vi "signalAnalysis.vi"(8 "error in (no error)":errorcluster, 9 "inpuPara":T1={"Rising[%] 1"=63.0, "Rising[%] 2"=99.0, "Falling[%]"=37.0}, 10 "data_scope":waveform(dbl), 11 "출력 전압 전류 특성":waveform(dbl)[](graph)=[{"t0"=timestamp(0 s since 1904-01-01), "dt"=0.0002, "Y"=array[10001 elements]}, {"t0"=timestamp(0 s since 1904-01-01), "dt"=0.0002, "Y"=array[10001 elements]}]) -> (0 "error out":errorcluster, 3 "data":T2)   [LabVIEW 2019]
uses:
  <vilib>/measure/mascope.llb/Transition Measurements 1 chan.vi
  <vilib>/measure/mascope.llb/Cycle Average and RMS 1 chan.vi
  <vilib>/measure/NI_MAPro.lvlib
panel:
  out "전체 저항 변화 2":waveform(dbl)(graph)
  out "measurement info":T3 {"ref levels"."ref units" items=["absolute", "relative"]; "ref levels"."high ref level" format="%.2p"; "ref levels"."low ref level" format="%.2p"; "ref levels"."mid ref level" format="%.2p"; "end time" format="%.2p"; "start time" format="%.2p"}
  out "접촉저항 변화":dbl[](graph)
  out "접촉 시 전압 변화":waveform(dbl)(graph)
  out "전체 저항 변화":dbl[](graph)
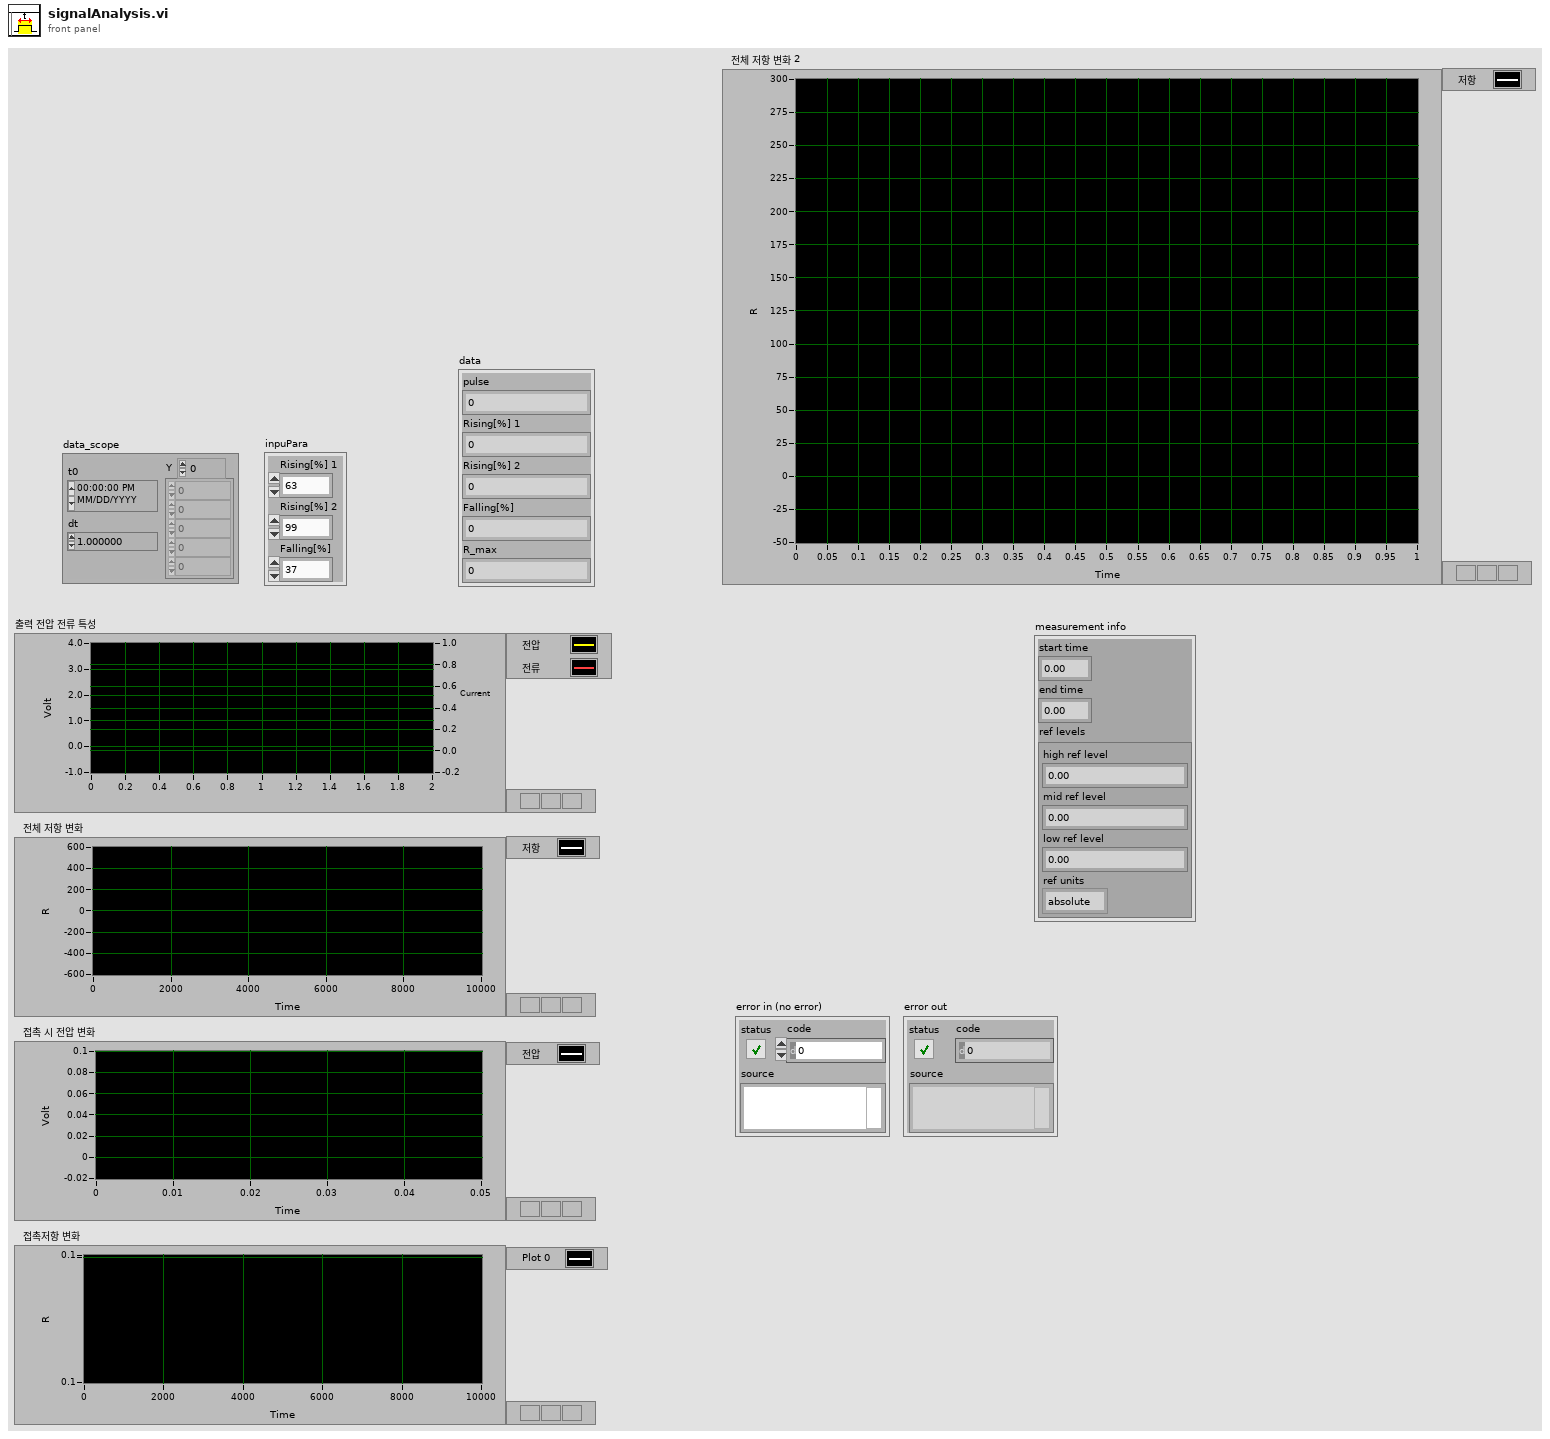
[diagram p1: front panel]
types:
  T1 = cluster{"Rising[%] 1":dbl, "Rising[%] 2":dbl, "Falling[%]":dbl}
  T2 = cluster{"pulse":i32, "Rising[%] 1":dbl, "Rising[%] 2":dbl, "Falling[%]":dbl, "R_max":dbl}
  T3 = cluster{"start time":dbl, "end time":dbl, "ref levels":cluster{"high ref level":dbl, "mid ref level":dbl, "low ref level":dbl, "ref units":u16}}
  T4 = cluster{"high ref level":dbl, "mid ref level":dbl, "low ref level":dbl, "ref units":u16}
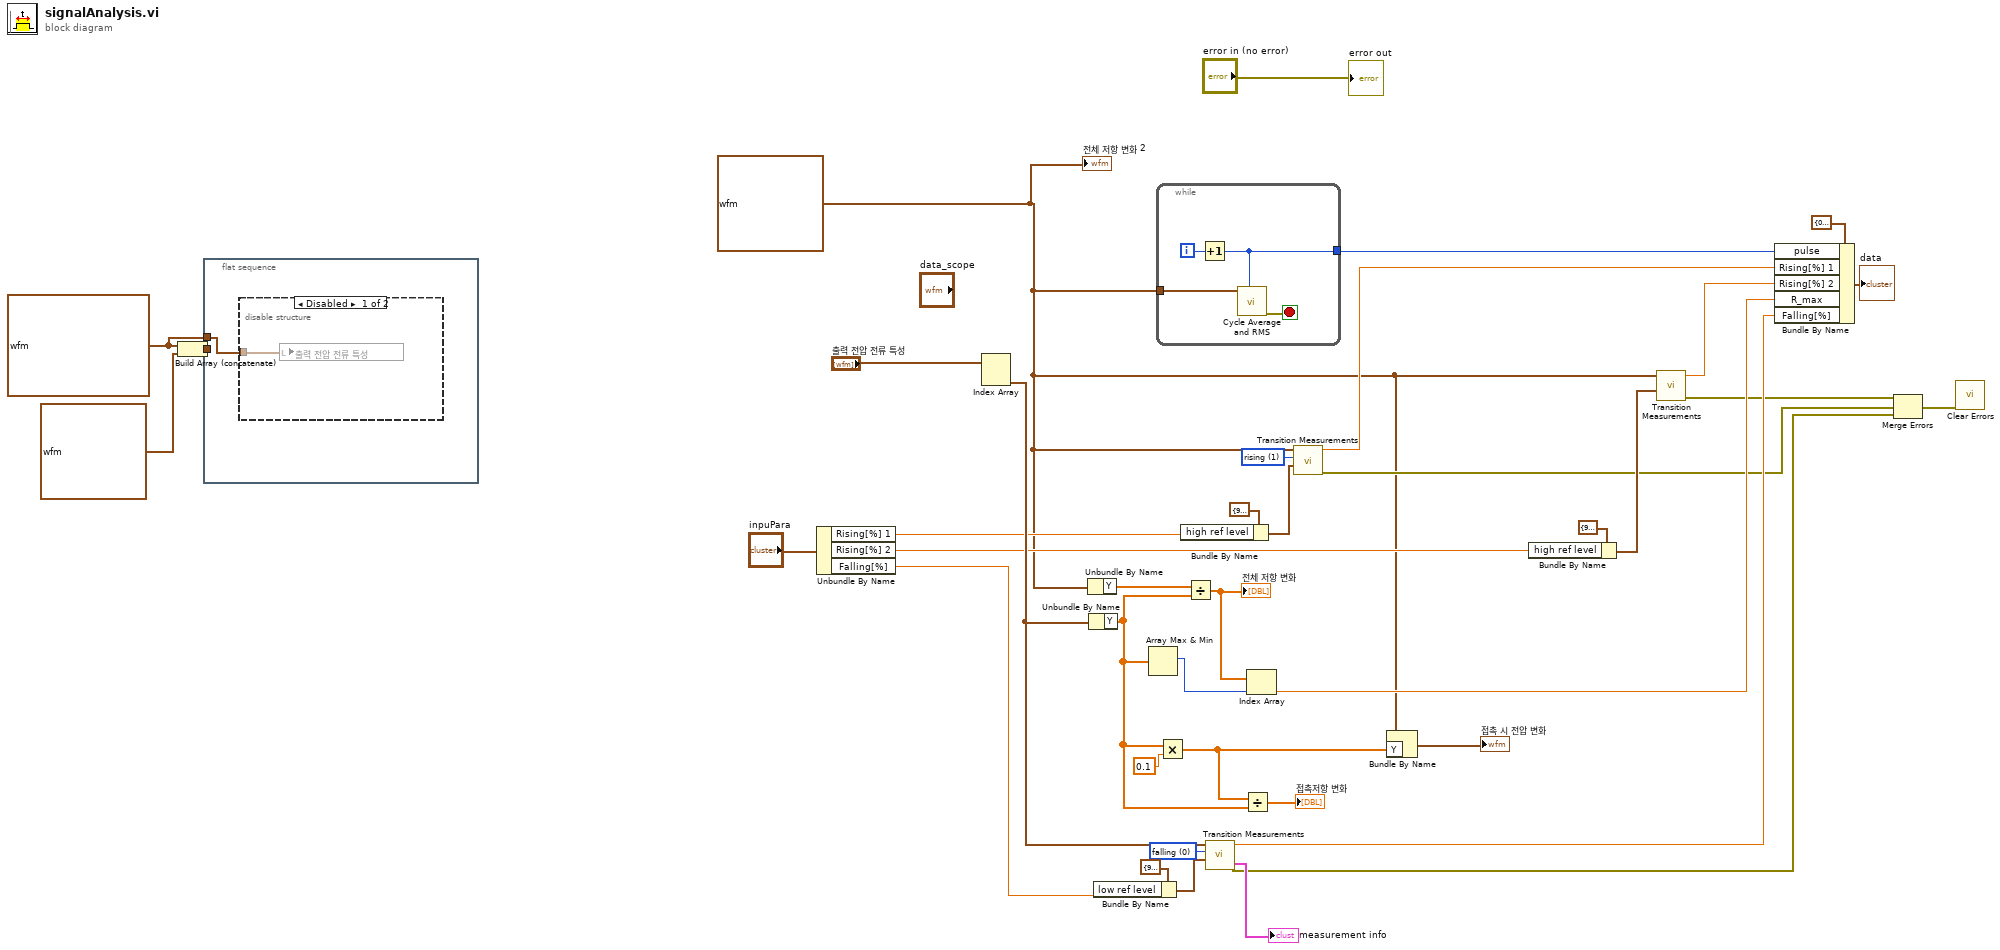
[diagram p0: block diagram]
diagram:
  w1 = waveform(dbl) {"t0"=timestamp(0 s since 1904-01-01), "dt"=5e-06, "Y"=array[200001 elements]} ("Waveform Graph")
  w18 = u16 1 items=["falling", "rising"] ("polarity (rising)")
  w20 = u16 0 items=["falling", "rising"] ("polarity (rising)")
  w28 = waveform(dbl)[] [{"t0"=timestamp(0 s since 1904-01-01), "dt"=0.0001, "Y"=array[20001 elements]}, {"t0"=timestamp(0 s since 1904-01-01), "dt"=0.0001, "Y"=array[20001 elements]}] ("Waveform Graph 2")
  n1 = Build Array (concatenate)(w28, waveform(dbl) {"t0"=timestamp(0 s since 1904-01-01), "dt"=0.0001, "Y"=array[20001 elements]} ("output waveform")) -> (w31:waveform(dbl)[])
  n2 = flat-sequence {
    tunnel: w31 -> [_]
    tunnel: w28 -> [w40]
    frame #0 {
      n3 = disable-structure shown="Disabled" {
        disable-tunnel: w40 -> [w41 _]
        frame Disabled {
          n4 = local write "출력 전압 전류 특성"(w41) -> ()
        }
        frame Enabled {
        }
      }
    }
  }
  n5 = Unbundle By Name("inpuPara") -> ("Rising[%] 1"=w9:dbl, "Rising[%] 2"=w8:dbl, "Falling[%]"=w7:dbl)
  n6 = Index Array(array="출력 전압 전류 특성") -> (element #2=w21:waveform(dbl))  [unwired: 2 in, 1 out]
  n7 = Unbundle By Name(w1) -> ("Y"=w35:dbl[])
  n8 = Unbundle By Name(w21) -> ("Y"=w27:dbl[])
  n9 = Bundle By Name(cluster=T4 {"high ref level"=90.0, "mid ref level"=50.0, "low ref level"=10.0, "ref units"=1} ("reference levels"), "low ref level"=w7) -> (w22:T4)
  n10 = Array Max & Min(array=w27) -> (max index (indices)=w33:i32)  [unwired: 3 out]
  n11 = while {
    tunnel: w1 -> [w45]
    tunnel: [w42] -> w17
    i -> [w44]
    stop <- w43 stop-if-true
    n12 = Increment(x=w44) -> (x+1=w42:i32)
    n13 = call-poly <vilib>:"Cycle Average and RMS.vi"("cycle number (1)"=w42, "signal in"=w45) -> ("error out"=w43:errorcluster)  [unwired: 6 in, 3 out]
  }
  n14 = Multiply(x=w27, y=0.1) -> (x*y=w26:dbl[])
  n15 = Bundle By Name(cluster=T4 {"high ref level"=90.0, "mid ref level"=50.0, "low ref level"=10.0, "ref units"=1} ("reference levels"), "high ref level"=w9) -> (w38:T4)
  n16 = Divide(x=w35, y=w27) -> (x/y=w34:dbl[])
  "전체 저항 변화" <- w34
  n17 = call-poly <vilib>:"Transition Measurements.vi"("reference levels"=w22, "polarity (rising)"=w20, "signal in"=w21) -> ("error out"=w3:errorcluster, "transition duration"=w14:dbl, "measurement info"=→"measurement info":T3)  [unwired: 3 in, 3 out]
  n18 = Divide(x=w26, y=w27) -> (x/y=→"접촉저항 변화":dbl[])
  n19 = Index Array(array=w34, index=w33) -> (element=w13:dbl)
  n20 = call-poly <vilib>:"Transition Measurements.vi"("reference levels"=w38, "polarity (rising)"=w18, "signal in"=w1) -> ("error out"=w4:errorcluster, "transition duration"=w16:dbl)  [unwired: 3 in, 4 out]
  n21 = Bundle By Name(cluster=w1, "Y"=w26) -> (→"접촉 시 전압 변화":waveform(dbl))
  n22 = Bundle By Name(cluster=T4 {"high ref level"=90.0, "mid ref level"=50.0, "low ref level"=10.0, "ref units"=1} ("reference levels"), "high ref level"=w8) -> (w37:T4)
  n23 = call-poly <vilib>:"Transition Measurements.vi"("reference levels"=w37, "signal in"=w1) -> ("error out"=w5:errorcluster, "transition duration"=w15:dbl)  [unwired: 4 in, 4 out]
  n24 = Bundle By Name(cluster=T2 {"pulse"=0, "Rising[%] 1"=0.0, "Rising[%] 2"=0.0, "Falling[%]"=0.0, "R_max"=0.0} ("data"), "pulse"=w17, "Rising[%] 1"=w16, "Rising[%] 2"=w15, "R_max"=w13, "Falling[%]"=w14) -> (→"data":T2)
  n25 = Merge Errors(w5, w4, w3) -> (w2:errorcluster)
  n26 = call <vilib>:"Clear Errors.vi"("error in (no error)"=w2) -> ()  [unwired: 5 in, 2 out]
  "error out" <- "error in (no error)"
  "전체 저항 변화 2" <- w1
